vi "TestRFGVRequests.vi"() -> ()   [LabVIEW 2015]
uses:
  TypeDef/RoomsActionEnum.ctl
panel:
  out "Remove":bool
  out "Add":bool
  out "Add Request 2":string
  out "Read Request 3":string
  out "Remove Request":string
  out "Add Request 1":string
  out "Read Requests 1":string
  out "Read Requests 2":string
  out "error out":errorcluster
  out "Pass":bool
  in  "Rooms":i32=101
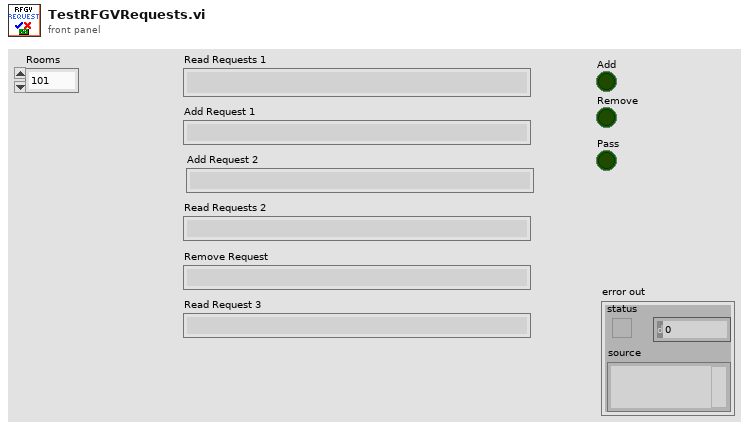
[diagram p1: front panel]
types:
  T1 = typedef "RoomsActionEnum.ctl" = enum16{"Init", "Add Room", "Remove Room", "Read Room", "Read Flag", "Read Flag State", "Write Flag State", "Read Flag Color", "Write Flag Color", "Read Bed Vacant", "Write Bed Vacant", "Read Personnel", "Add Personnel", "Remove Personnel", "Read Requests", "Add Request", "Remove Request", "Read Beacon ID", "Write Beacon ID", "Write Bed URL", "Read Bed URL", "Read Rooms Numbers", "Write Flag"}
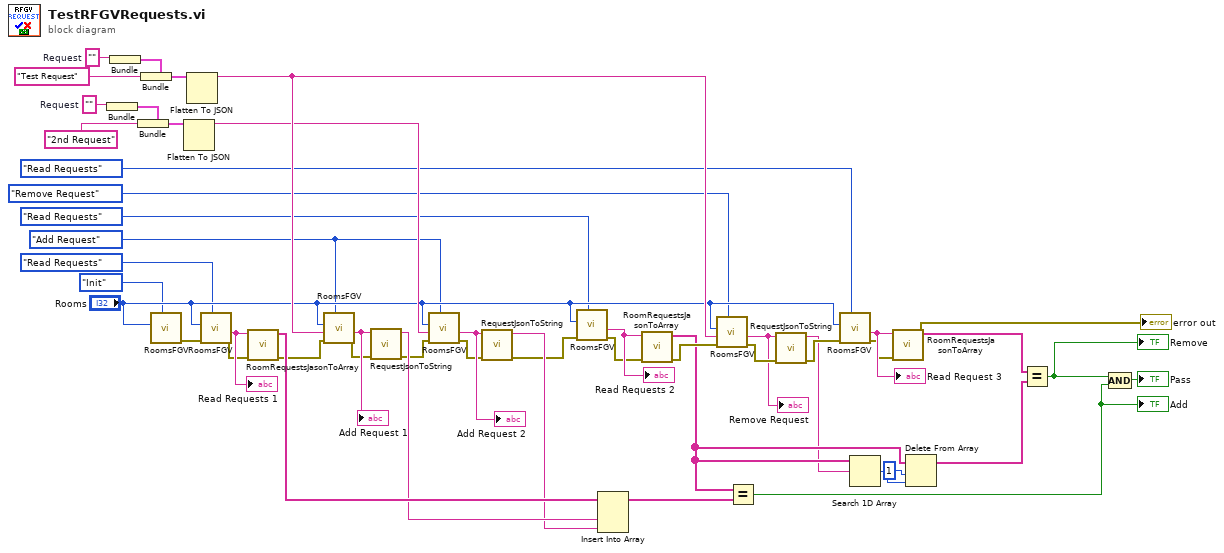
[diagram p0: block diagram]
diagram:
  w4 = RoomsActionEnum."Add Request" ("Actions")
  w38 = ""  # Request
  w48 = ""  # Request
  n1 = Bundle("Request"=w38) -> (w39:cluster{"Request":string})  [unwired: 1 in]
  n2 = Bundle("Request"=w48) -> (w47:cluster{"Request":string})  [unwired: 1 in]
  n3 = Bundle(cluster=w39, "Request"="2nd Request" ("Request 2")) -> (w40:cluster{"Request":string})
  n4 = Bundle(cluster=w47, "Request"="Test Request") -> (w46:cluster{"Request":string})
  n5 = call "RoomsFGV.vi"("Actions"=RoomsActionEnum."Init", "Room"="Rooms") -> ("error out"=w49:errorcluster)  [unwired: 8 in, 1 out]
  n6 = Flatten To JSON(anything=w40) -> (JSON string=w37:string)  [unwired: 2 in, 1 out]
  n7 = Flatten To JSON(anything=w46) -> (JSON string=w45:string)  [unwired: 2 in, 1 out]
  n8 = call "RoomsFGV.vi"("Actions"=RoomsActionEnum."Read Requests", "error in (no error)"=w49, "Room"="Rooms") -> ("error out"=w28:errorcluster, "Data Out"=w34:string)  [unwired: 7 in]
  "Read Requests 1" <- w34
  n9 = call "RoomRequestsJasonToArray.vi"("error in (no error)"=w28, "Data Out"=w34) -> ("error out"=w27:errorcluster, "REQs"=w33:string[])  [unwired: 8 in]
  n10 = call "RoomsFGV.vi"("Actions"=w4, "error in (no error)"=w27, "Data In"=w45, "Room"="Rooms") -> ("error out"=w26:errorcluster, "Data Out"=w36:string)  [unwired: 6 in]
  "Add Request 1" <- w36
  n11 = call "RequestJsonToString.vi"("error in (no error)"=w26, "Data Out"=w36) -> ("error out"=w25:errorcluster, "Request"=w32:string)  [unwired: 8 in]
  n12 = call "RoomsFGV.vi"("Actions"=w4, "error in (no error)"=w25, "Data In"=w37, "Room"="Rooms") -> ("error out"=w24:errorcluster, "Data Out"=w35:string)  [unwired: 6 in]
  "Add Request 2" <- w35
  n13 = call "RequestJsonToString.vi"("error in (no error)"=w24, "Data Out"=w35) -> ("error out"=w23:errorcluster, "Request"=w31:string)  [unwired: 8 in]
  n14 = call "RoomsFGV.vi"("Actions"=RoomsActionEnum."Read Requests", "error in (no error)"=w23, "Room"="Rooms") -> ("error out"=w22:errorcluster, "Data Out"=w30:string)  [unwired: 7 in]
  "Read Requests 2" <- w30
  n15 = Insert Into Array(array=w33, new element #1=w32, new element #2=w31) -> (w29:string[])  [unwired: 1 in]
  n16 = call "RoomRequestsJasonToArray.vi"("error in (no error)"=w22, "Data Out"=w30) -> ("error out"=w21:errorcluster, "REQs"=w15:string[])  [unwired: 8 in]
  n17 = call "RoomsFGV.vi"("Actions"=RoomsActionEnum."Remove Request", "error in (no error)"=w21, "Data In"=w45, "Room"="Rooms") -> ("error out"=w20:errorcluster, "Data Out"=w18:string)  [unwired: 6 in]
  "Remove Request" <- w18
  n18 = Equal?(x=w15, y=w29) -> (x = y?=w43:bool)
  "Add" <- w43
  n19 = call "RequestJsonToString.vi"("error in (no error)"=w20, "Data Out"=w18) -> ("error out"=w19:errorcluster, "Request"=w14:string)  [unwired: 8 in]
  n20 = call "RoomsFGV.vi"("Actions"=RoomsActionEnum."Read Requests", "error in (no error)"=w19, "Room"="Rooms") -> ("error out"=w12:errorcluster, "Data Out"=w13:string)  [unwired: 7 in]
  "Read Request 3" <- w13
  n21 = Search 1D Array(1D array=w15, element=w14) -> (index of element=w17:i32)  [unwired: 1 in]
  n22 = call "RoomRequestsJasonToArray.vi"("error in (no error)"=w12, "Data Out"=w13) -> ("error out"=→"error out":errorcluster, "REQs"=w10:string[])  [unwired: 8 in]
  n23 = Delete From Array(array=w15, length=1, index=w17) -> (array with subset deleted=w9:string[])  [unwired: 1 out]
  n24 = Equal?(x=w10, y=w9) -> (x = y?=w44:bool)
  "Remove" <- w44
  n25 = Compound Arithmetic op=AND(w44, w43) -> (→"Pass":bool)
